vi "Test TEC.vi"() -> ()   [LabVIEW 2012]
uses:
  Devices/TE Cooler/TE Cooler.lvclass
panel:
  out "Power (%)":sgl
  out "T1":sgl
  out "error out 2":errorcluster
  out "error out":errorcluster={"status"=TRUE, "code"=-1073807339, "source"="VISA Read in Serial IO.lvclass:Cmd to R_W - Synchronous.vi->TE Cooler.lvlib:TE Cooler.lvclass:Write to Port.vi->TE Cooler.lvlib:TE Cooler.lvclass:Init.vi->cPAS.lvclass:Serial Config.vi->cPAS.lvclass:Start Config.vi->PAS.lvclass:Configure.vi->PAS Server.vi->Combined Server.vi"}
  in  "Boolean":bool
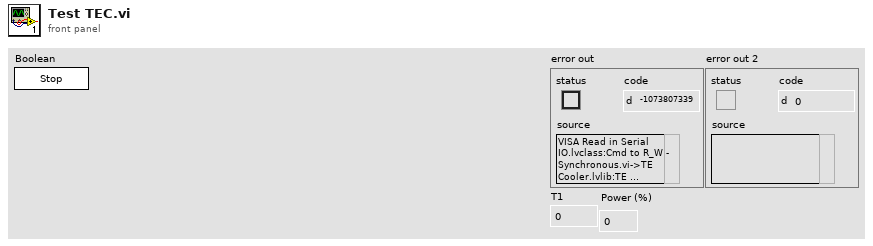
[diagram p1: front panel]
types:
  T1 = cluster{"baud rate (9600)":u32, "data bits (8)":u16, "stop bits (10: 1 bit)":u16, "parity (0:none)":enum16{"None", "Odd", "Even", "Mark", "Space"}, "flow control (0:none)":u16, "endModeforReads":u16, "endModeforWrites":u16}
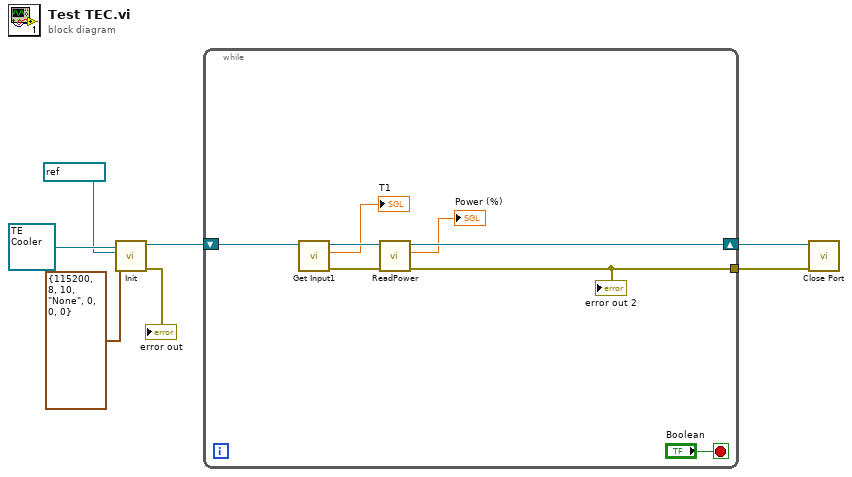
[diagram p0: block diagram]
diagram:
  n1 = call-dynamic "Init.vi"("serialCfg"=T1 {"baud rate (9600)"=115200, "data bits (8)"=8, "stop bits (10: 1 bit)"=10, "parity (0:none)"=enum."None", "flow control (0:none)"=0, "endModeforReads"=0, "endModeforWrites"=0}, "Port"=refnum<visa-resource-name> "COM2", "TE Cooler in"=refnum<class "TE Cooler.lvclass"> refnum ("TE Cooler.lvlib:TE Cooler.lvclass")) -> ("error out"=→"error out":errorcluster, "TE Cooler out"=w6:refnum<class "TE Cooler.lvclass">)  [unwired: 7 in]
  n2 = while {
    shift-right: [w13] -> w5
    shift-left: w6 -> [w15]
    tunnel: [w12] -> w3
    stop <- "Boolean" stop-if-true
    n3 = call "Get Input1.vi"("TE Cooler in"=w15) -> ("error out"=w11:errorcluster, "T1"=→"T1":sgl, "TE Cooler out"=w14:refnum<class "TE Cooler.lvclass">)  [unwired: 8 in]
    n4 = call "ReadPower.vi"("error in"=w11, "TE Cooler in"=w14) -> ("error out"=w12:errorcluster, "Power (%)"=→"Power (%)":sgl, "TE Cooler out"=w13:refnum<class "TE Cooler.lvclass">)  [unwired: 7 in]
    "error out 2" <- w12
  }
  n5 = call-dynamic "Close Port.vi"("error in (no error)"=w3, "Serial IO in"=w5) -> ()  [unwired: 8 in, 2 out]
